vi "Test.Runner.kria.bats.parser.vi"() -> ()   [LabVIEW 2020]
uses:
  <vilib>/rvi/interface/nirviOpenFPGA/nirviOpenFPGA.xnode
  <vilib>/rvi/interface/nirviMethod/nirviMethod.xnode
  <vilib>/rvi/interface/nirviCloseFPGA/nirviCloseFPGA.xnode
  <vilib>/rvi/errors/niLvFpgaMergeErrorWithErrorCode.vi
  <vilib>/FPGAPlugInAG/Dynamic/niLvFpga_ReadFifo_Dynamic.vi
  <vilib>/rvi/interface/nirviReadWriteControl/nirviReadWriteControl.xnode
  <vilib>/rvi/interface/Simulation/niFpgaSimulationCallBeginRW.vi
  <vilib>/rvi/errors/niLvFpgaAdjustHostInterfaceError.vi
  submodules/Market.Data.Common/host/fpganow.common.host.lvlib
  NiFpgaLv.dll
  <vilib>/Utility/error.llb/Error Cluster From Error Code.vi
  <vilib>/FPGAPlugInAG/Dynamic/niLvFpga_Run_Dynamic.vi
  <vilib>/FPGAPlugInAG/Dynamic/niLvFpga_WriteFifo_Dynamic.vi
  <vilib>/FPGAPlugInAG/Dynamic/niLvFpga_Close_Dynamic.vi
  FPGA Bitfiles/market.data.poc_FPGATarget_poc.ip.kria_VbtSJiBgbQ0.lvbitx
  fpga/poc.ip.kria.vi
  <vilib>/FPGAPlugInAG/USRP-X410/niLvFpga_Open_USRP-X410.vi
  <vilib>/rvi/interface/common/dynamic/niFpgaDynamicAddResources.vi
  submodules/Market.Data.Common/fpga/orderbook.command.type.ctl
  submodules/Market.Data.Common/fpga/fpganow.common.fpga.lvlib
  submodules/Market.Data.Common/fpga/orderbook.command.ctl
panel:
  out "MDebug":u64[][](array[numeric]) format="%.0x"
  out "Ob.cmd [str]":string[](array[string])
  out "Data Sent 3":u64[][](array[numeric]) format="%016x"
  out "Debug":u64[][](array[numeric]) format="%.0x"
  out "Deserialized\nOrderBook.Commands":u64[](array[numeric]) format="%.0x"
  out "OrderBook.Command[]":T1[](array[typedef]) {"price" format="%.0x"; "symbol" format="%.0x"; "orderId" format="%.0x"; "side" format="%.0x"}
  out "error out":errorcluster
  in  "error in":errorcluster
  in  "Raw_Data File Path":path=path "C:/work/fpganow/Market.Data.PoC/cboe_pitch/generated_2025_05_02.pcap"
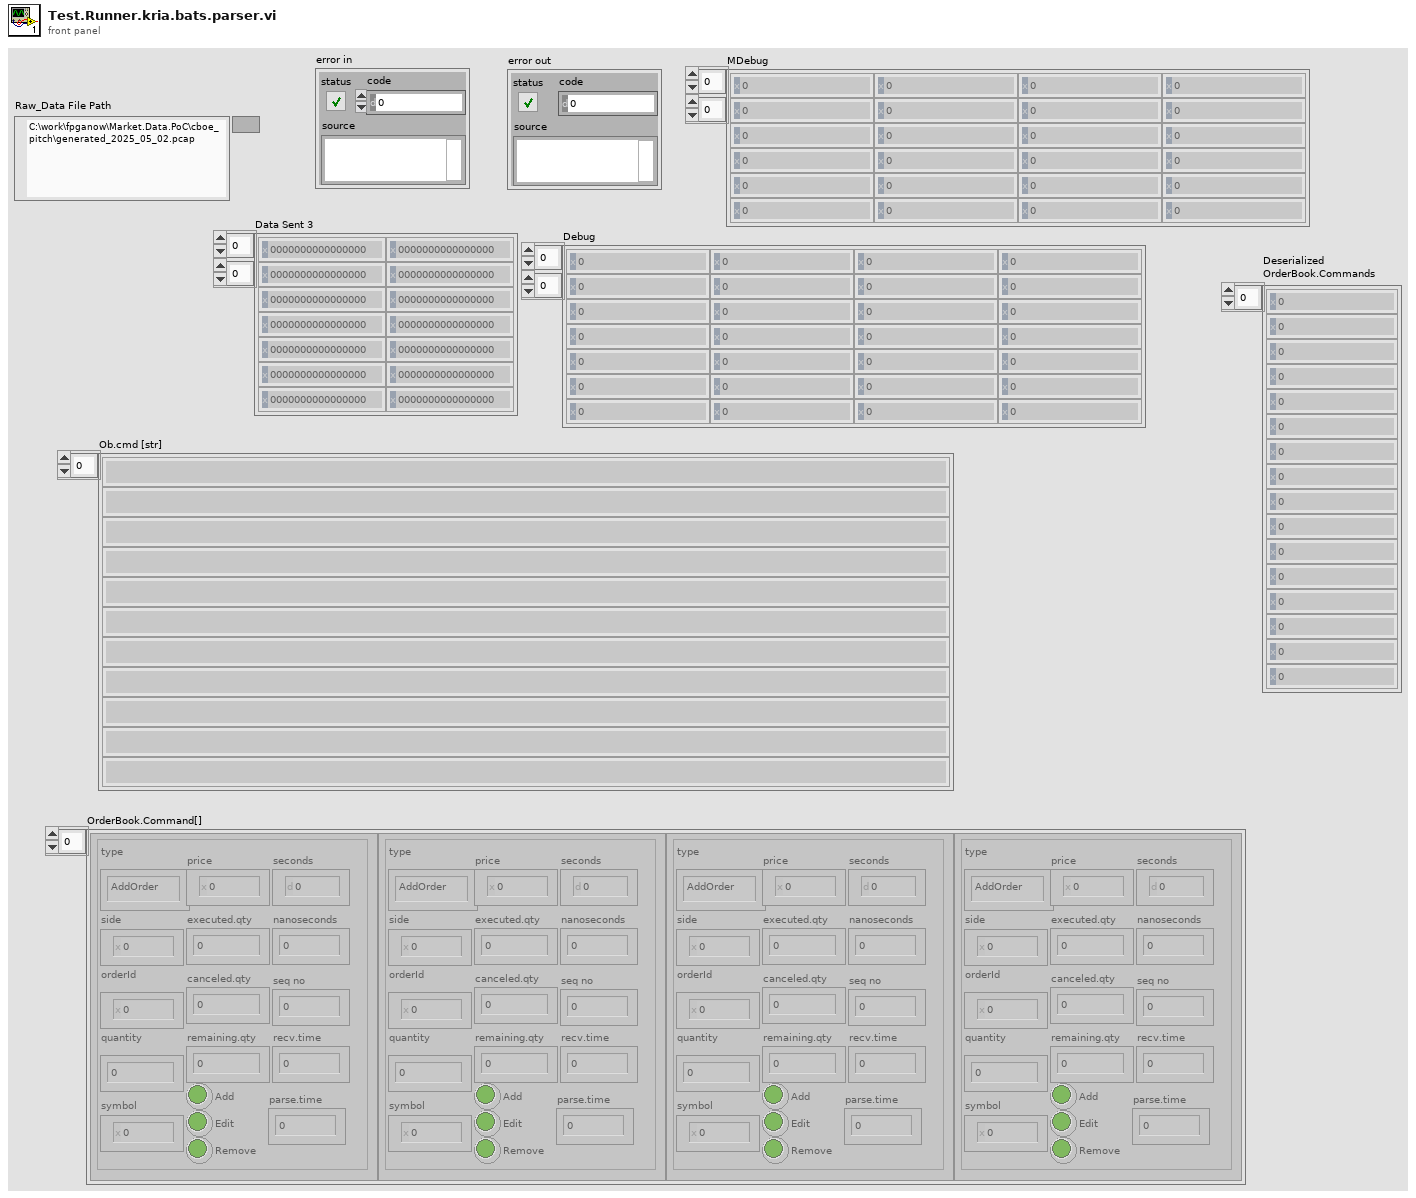
[diagram p1: front panel]
types:
  T1 = typedef "fpganow.common.fpga.lvlib/orderbook.command.ctl" = cluster{"type":T2, "side":u8, "orderId ":u64, "quantity":u32, "symbol":u64, "price":u64, "executed.qty":u32, "canceled.qty":u32, "remaining.qty":u32, "seconds":u64, "nanoseconds":u64, "Add":bool, "Edit":bool, "Remove":bool, "seq no":u32, "recv.time":u64, "parse.time":u64}
  T2 = typedef "fpganow.common.fpga.lvlib/orderbook.command.type.ctl" = enum8{"Time", "AddOrder", "OrderExecuted", "OrderExecutedAtPrice", "ReduceSize", "ModifyOrder", "DeleteOrder", "Get.Everything", "Get.All.Orders", "Get.Top"}
  T3 = typedef "record.ctl" = cluster{"ts_sec":u32, "ts_usec":u32, "incl_len":u32, "orig_len":u32, "payload":u8[]}
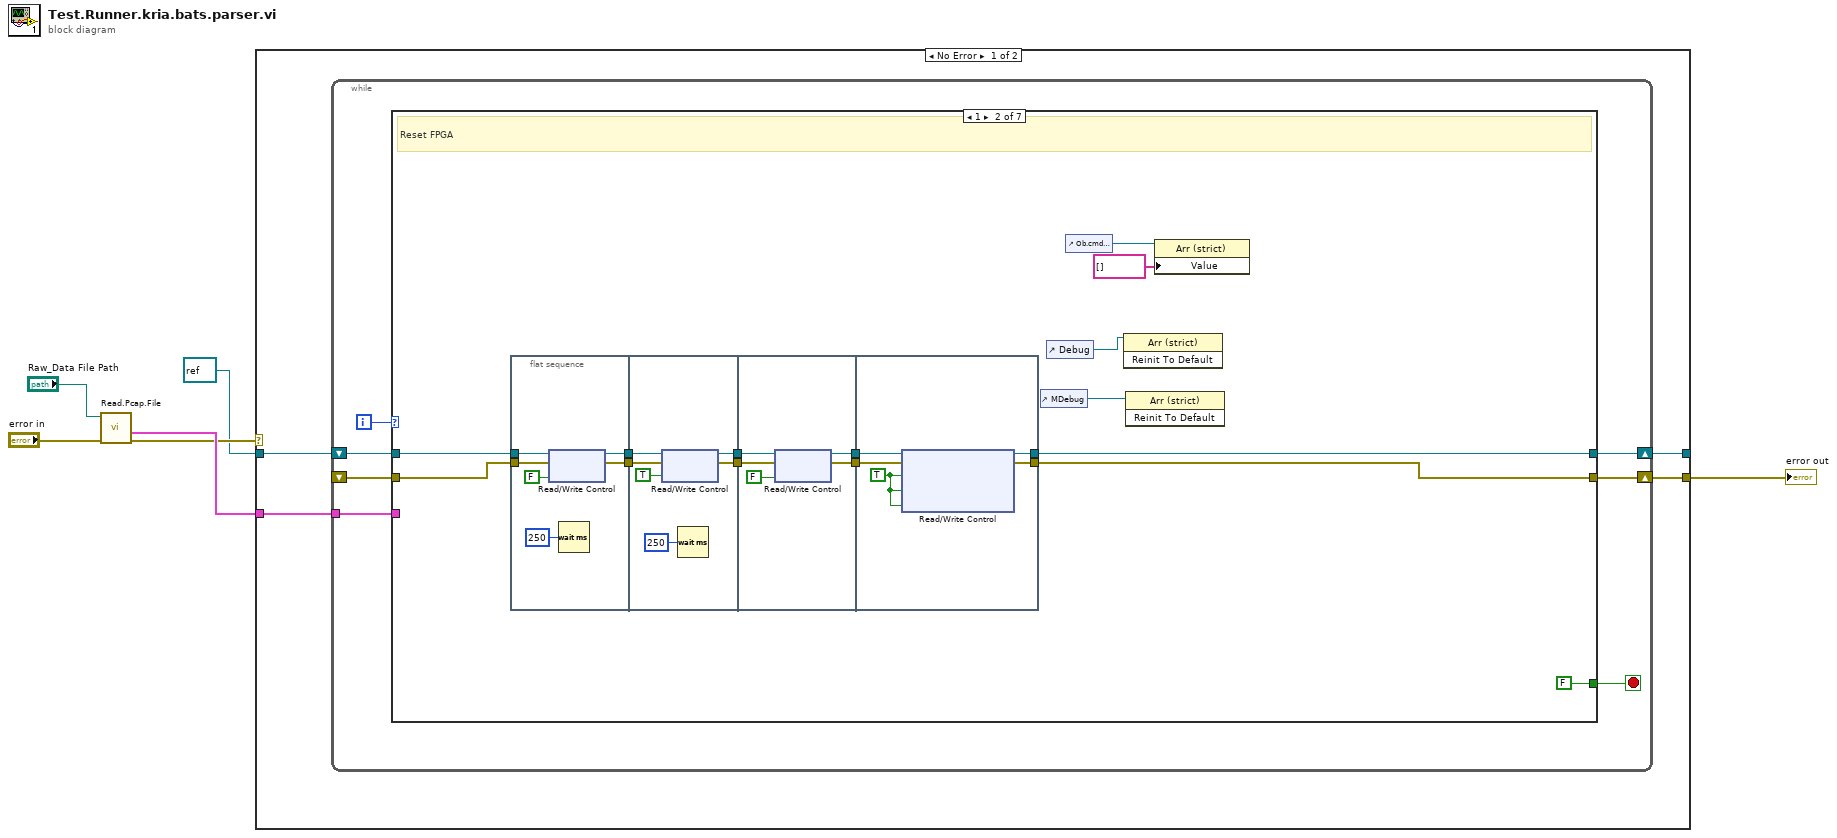
[diagram p0: block diagram]
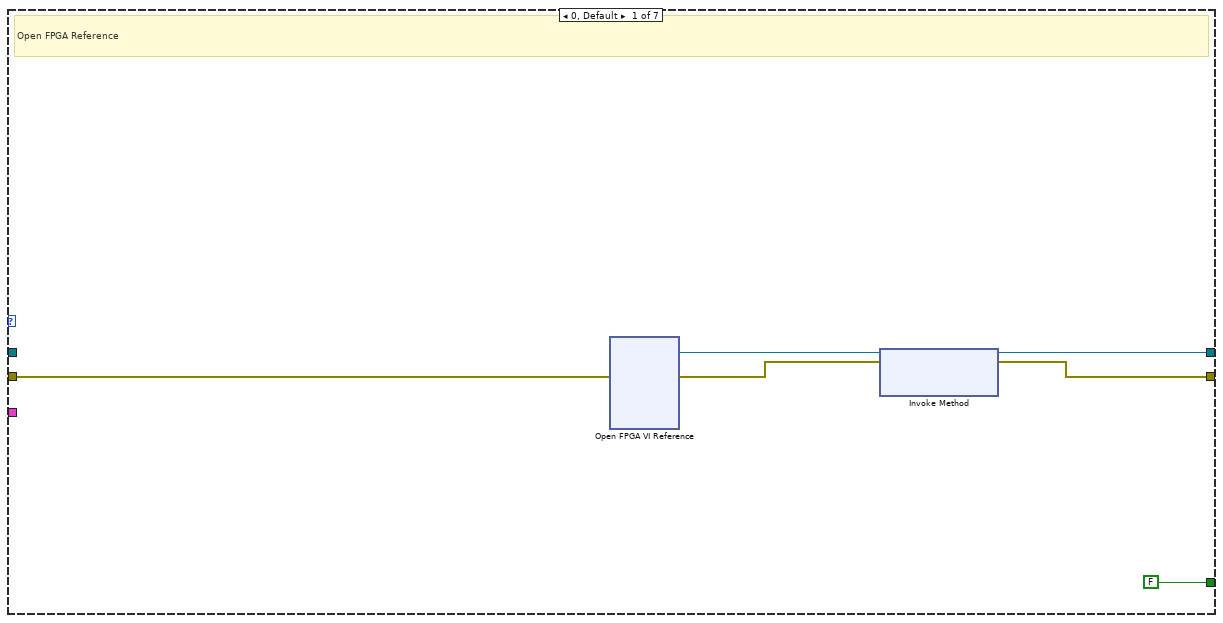
[diagram p2: hidden frame]
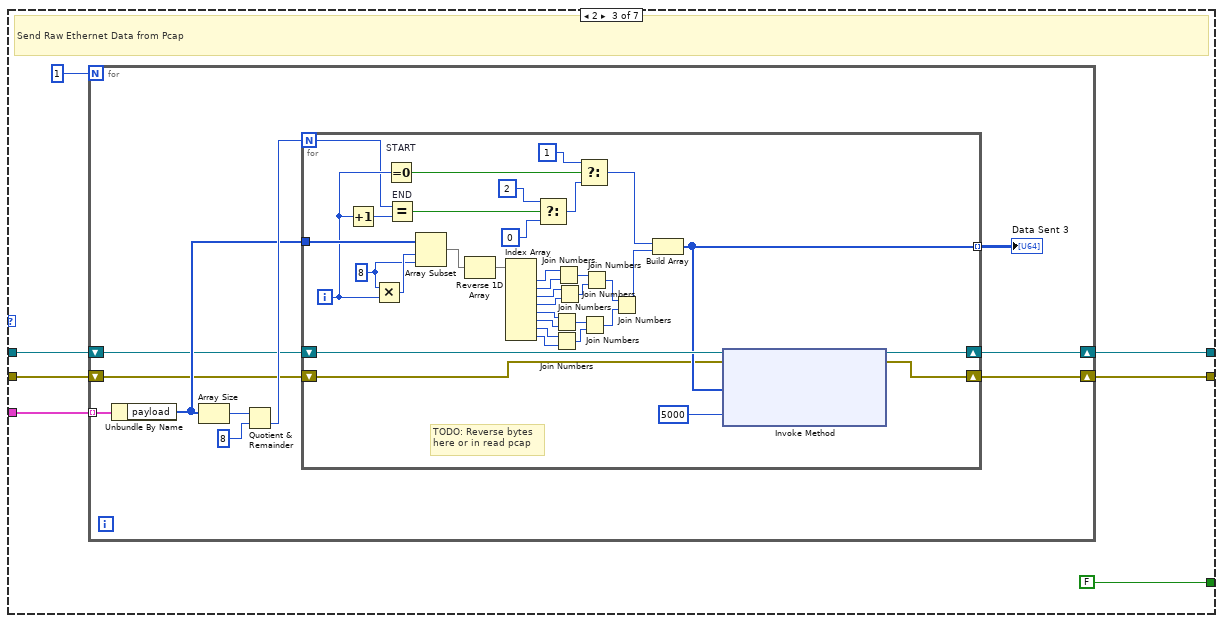
[diagram p3: hidden frame]
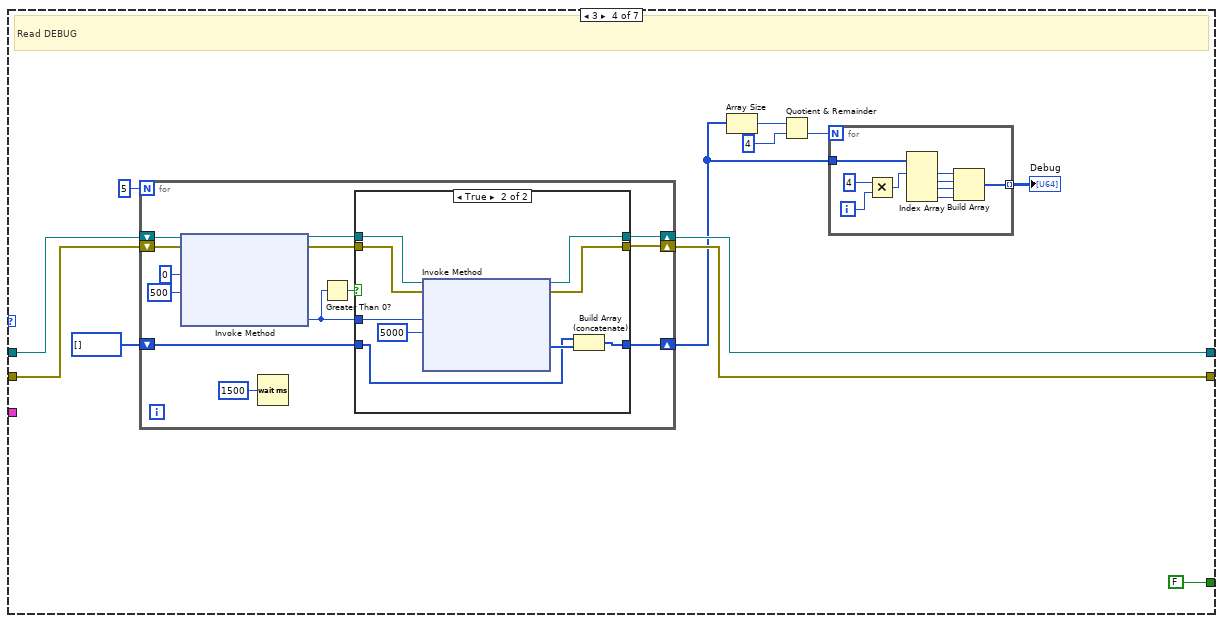
[diagram p4: hidden frame]
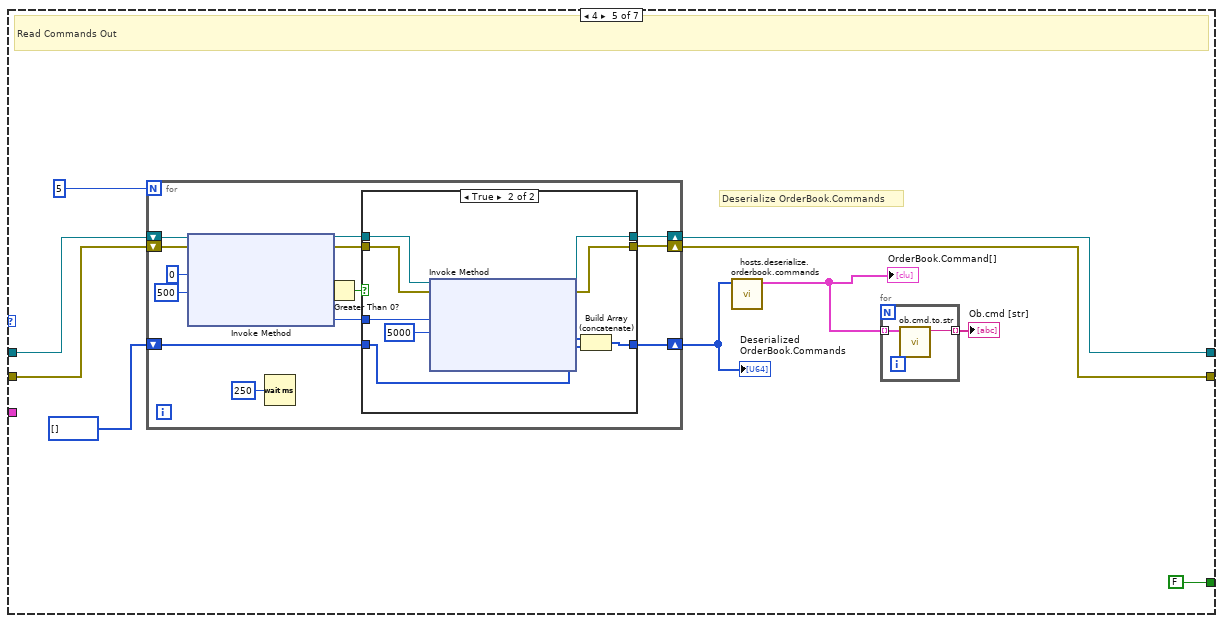
[diagram p6: hidden frame]
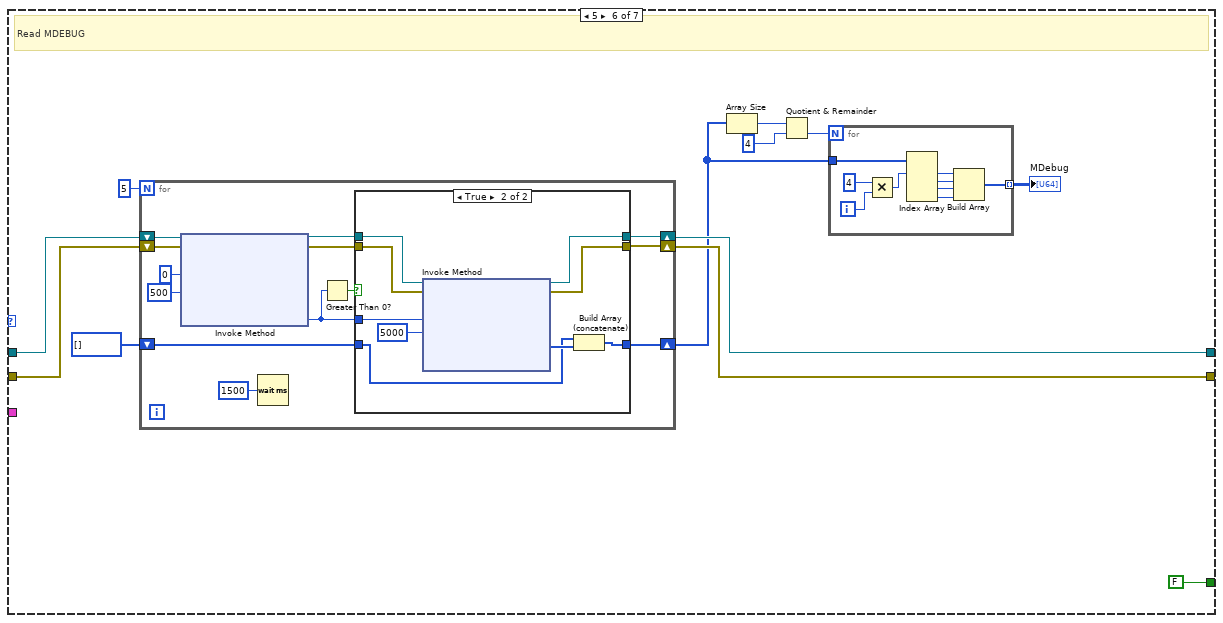
[diagram p8: hidden frame]
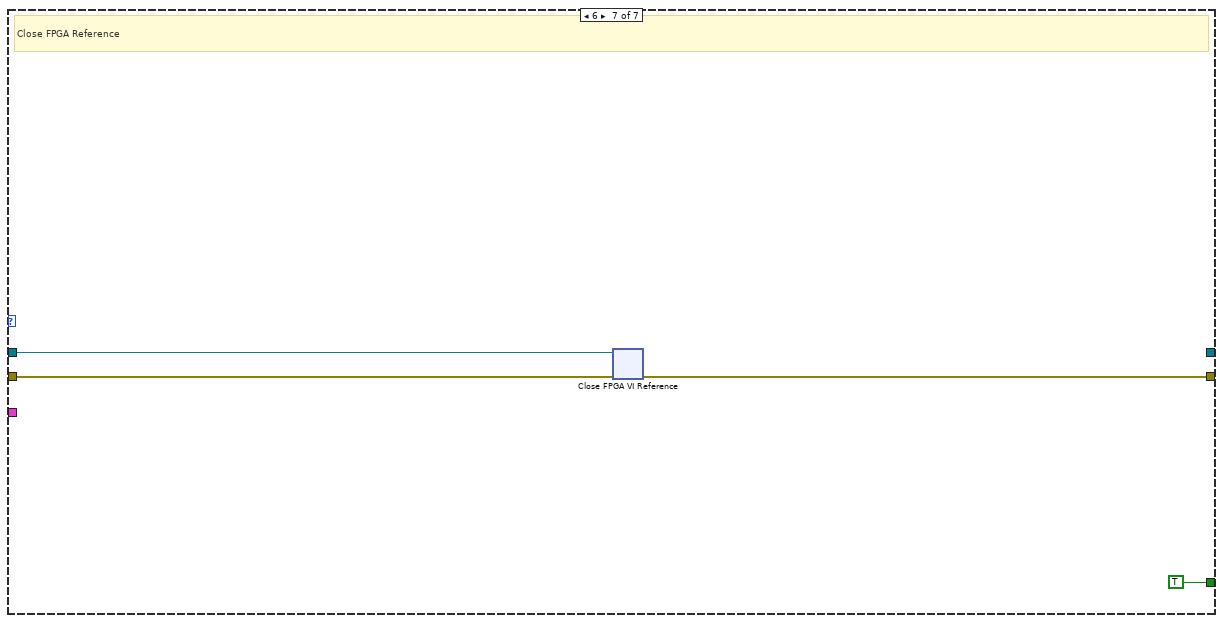
[diagram p10: hidden frame]
diagram:
  n1 = call "Read.Pcap.File.vi"("error in"="error in", "Path"="Raw_Data File Path") -> ("error out"=w4:errorcluster, "Records"=w5:T3[])  [unwired: 6 in, 2 out]
  n2 = case shown="No Error" w4 {
    selector: w4 -> [_ w247]
    tunnel: w5 -> [w10 _]
    tunnel: refnum<k20> refnum ("FPGA VI Reference Out") -> [w9 _]
    tunnel: [w8 _] -> _
    tunnel: [w7 w247] -> w3
    frame No Error {
      n3 = while {
        tunnel: w10 -> [w17]
        shift-right: [w11] -> w8
        shift-left: w9 -> [w16]
        shift-right: [w15] -> w7
        shift-left: _ -> [w14]
        i -> [w13]
        stop <- w12 stop-if-true
        n4 = case shown="1" w13 {
          tunnel: w17 -> [_ _ w62 _ _ _ _]
          tunnel: w16 -> [_ w38 w67 w125 w168 w208 w246]
          tunnel: [w19 w37 w66 w122 w165 w205 _] -> w11
          tunnel: [w18 w36 w65 w121 w164 w204 w244] -> w15
          tunnel: w14 -> [w22 w35 w64 w123 w166 w206 w245]
          tunnel: [FALSE FALSE FALSE FALSE FALSE FALSE TRUE] -> w12
          frame 0, Default {
            # "Open FPGA Reference"
            n5 = xnode "Open FPGA VI Reference"("error in"=w22) -> ("FPGA VI Reference Out"=w21:refnum<k20>, "error out"=w20:errorcluster)  [unwired: 1 in]
            n6 = xnode "Invoke Method"("FPGA VI Reference In"=w21, "error in"=w20) -> ("FPGA VI Reference Out"=w19:refnum<k20>, "error out"=w18:errorcluster)  [unwired: 1 in]
          }
          frame 1 {
            # "Reset FPGA"
            n7 = flat-sequence {
              tunnel: w38 -> [w44]
              tunnel: w35 -> [w41]
              tunnel: [w43] -> w33
              tunnel: [w42] -> w32
              tunnel: w33 -> [w49]
              tunnel: w32 -> [w50]
              tunnel: [w47] -> w31
              tunnel: [w48] -> w30
              tunnel: w31 -> [w54]
              tunnel: w30 -> [w55]
              tunnel: [w52] -> w25
              tunnel: [w53] -> w24
              tunnel: [w58] -> w36
              tunnel: [w57] -> w37
              tunnel: w25 -> [w59]
              tunnel: w24 -> [w60]
              frame #0 {
                n8 = xnode "Read/Write Control"("FPGA VI Reference In"=w44, "error in"=w41, "ip.reset"=FALSE ("Reset")) -> ("FPGA VI Reference Out"=w43:refnum<k20>, "error out"=w42:errorcluster)
                n9 = Wait (ms)(milliseconds to wait=u32 250) -> ()  [unwired: 1 out]
              }
              frame #1 {
                n10 = xnode "Read/Write Control"("FPGA VI Reference In"=w49, "error in"=w50, "ip.reset"=TRUE ("Reset")) -> ("FPGA VI Reference Out"=w47:refnum<k20>, "error out"=w48:errorcluster)
                n11 = Wait (ms)(milliseconds to wait=u32 250) -> ()  [unwired: 1 out]
              }
              frame #2 {
                n12 = xnode "Read/Write Control"("FPGA VI Reference In"=w54, "error in"=w55, "ip.reset"=FALSE ("Reset")) -> ("FPGA VI Reference Out"=w52:refnum<k20>, "error out"=w53:errorcluster)
              }
              frame #3 {
                w56 = TRUE ("MDEBUG.TREADY")
                n13 = xnode "Read/Write Control"("FPGA VI Reference In"=w59, "error in"=w60, "MDEBUG.TREADY"=w56, "CMD.TREADY"=w56, "DEBUG.TREADY"=w56) -> ("FPGA VI Reference Out"=w57:refnum<k20>, "error out"=w58:errorcluster)
              }
            }
            n14 = control-ref of="MDebug"() -> (w29:refnum<vi>)
            n15 = control-ref of="Debug"() -> (w28:refnum<vi>)
            n16 = control-ref of="Ob.cmd [str]"() -> (w27:refnum<vi>)
            n17 = invoke class="Arr (strict)" method="Reinit To Default"(reference=w28) -> ()  [unwired: 2 in, 3 out]
            n18 = invoke class="Arr (strict)" method="Reinit To Default"(reference=w29) -> ()  [unwired: 2 in, 3 out]
            n19 = property class="Arr (strict)"(reference=w27, "Value"=string[] []) -> ()  [unwired: 1 in, 2 out]
          }
          frame 2 {
            # "Send Raw Ethernet Data from Pcap"
            n20 = for {
              N: 1 -> [_]
              tunnel: w62 -> [w73] mode=indexing
              shift-right: [w71] -> w66
              shift-left: w67 -> [w70]
              shift-right: [w69] -> w65
              shift-left: w64 -> [w68]
              n21 = Unbundle By Name(w73) -> ("payload"=w74:u8[])
              n22 = Array Size(array=w74) -> (size(s)=w77:i32)
              n23 = Quotient & Remainder(x=w77, y=8) -> (floor(x/y)=w75:i32)  [unwired: 1 out]
              n24 = for {
                N: w75 -> [w109]
                tunnel: w74 -> [w111]
                tunnel: [w83] -> w72 mode=indexing
                shift-right: [w85] -> w71
                shift-left: w70 -> [w84]
                shift-right: [w81] -> w69
                shift-left: w68 -> [w80]
                i -> [w110]
                w112 = 8 ("x")
                # "TODO: Reverse bytes\nhere or in read pcap"
                n25 = Increment(x=w110) -> (x+1=w108:i32)
                n26 = Multiply(x=w112, y=w110) -> (x*y=w113:i32)
                n27 = Equal To 0? "START"(x=w110) -> (x = 0?=w107:bool)
                n28 = Equal? "END"(x=w109, y=w108) -> (x = y?=w105:bool)
                n29 = Array Subset(array=w111, index=w113, length=w112) -> (w78:u8[])
                n30 = Reverse 1D Array(array=w78) -> (reversed array=w79:u8[])
                n31 = Index Array(array=w79) -> (element #1=w100:u8, element #2=w101:u8, element #3=w99:u8, element #4=w98:u8, element #5=w96:u8, element #6=w97:u8, element #7=w95:u8, element #8=w94:u8)  [unwired: 8 in]
                n32 = Select(t=u64 2, s=w105, f=u64 0) -> (s? t:f=w102:u64)
                n33 = Join Numbers(hi=w96, lo=w97) -> ((hi.lo)=w91:u16)
                n34 = Join Numbers(hi=w95, lo=w94) -> ((hi.lo)=w90:u16)
                n35 = Join Numbers(hi=w100, lo=w101) -> ((hi.lo)=w93:u16)
                n36 = Join Numbers(hi=w99, lo=w98) -> ((hi.lo)=w92:u16)
                n37 = Select(t=u64 1, s=w107, f=w102) -> (s? t:f=w86:u64)
                n38 = Join Numbers(hi=w91, lo=w90) -> ((hi.lo)=w88:u32)
                n39 = Join Numbers(hi=w93, lo=w92) -> ((hi.lo)=w89:u32)
                n40 = Join Numbers(hi=w89, lo=w88) -> ((hi.lo)=w87:u64)
                n41 = Build Array(w86, w87) -> (w83:u64[])
                n42 = xnode "Invoke Method"("FPGA VI Reference In"=w84, "error in"=w80, "Data"=w83, "Timeout (ms)"=5000) -> ("FPGA VI Reference Out"=w85:refnum<k20>, "error out"=w81:errorcluster)  [unwired: 1 out]
              }
              "Data Sent 3" <- w72
            }
          }
          frame 3 {
            # "Read DEBUG"
            n43 = for {
              N: 5 -> [_]
              shift-right: [w141] -> w122
              shift-left: w125 -> [w147]
              shift-right: [w140] -> w121
              shift-left: w123 -> [w146]
              shift-right: [w142] -> w117
              shift-left: u64[] [] -> [w136]
              n44 = xnode "Invoke Method"("FPGA VI Reference In"=w147, "error in"=w146, "Number of Elements"=u32 0, "Timeout (ms)"=500) -> ("FPGA VI Reference Out"=w139:refnum<k20>, "error out"=w138:errorcluster, "Elements Remaining"=w137:u32)  [unwired: 1 out]
              n45 = Wait (ms)(milliseconds to wait=u32 1500) -> ()  [unwired: 1 out]
              n46 = Greater Than 0?(x=w137) -> (x > 0?=w143:bool)
              n47 = case shown="True" w143 {
                tunnel: [w148 w158] -> w142
                tunnel: [w150 w157] -> w141
                tunnel: [w149 w156] -> w140
                tunnel: w139 -> [w150 w155]
                tunnel: w138 -> [w149 w154]
                tunnel: w137 -> [_ w153]
                tunnel: w136 -> [w148 w151]
                frame False {
                }
                frame True {
                  n48 = xnode "Invoke Method"("FPGA VI Reference In"=w155, "error in"=w154, "Number of Elements"=w153, "Timeout (ms)"=5000) -> ("FPGA VI Reference Out"=w157:refnum<k20>, "error out"=w156:errorcluster, "Data"=w159:u64[])  [unwired: 1 out]
                  n49 = Build Array (concatenate)(w151, w159) -> (w158:u64[])
                }
              }
            }
            n50 = Array Size(array=w117) -> (size(s)=w119:i32)
            n51 = Quotient & Remainder(x=w119, y=4) -> (floor(x/y)=w115:i32)  [unwired: 1 out]
            n52 = for {
              N: w115 -> [_]
              tunnel: w117 -> [w134]
              tunnel: [w126] -> w116 mode=indexing
              i -> [w133]
              n53 = Multiply(x=4, y=w133) -> (x*y=w132:i32)
              n54 = Index Array(array=w134, index #1=w132) -> (element #1=w130:u64, element #2=w127:u64, element #3=w128:u64, element #4=w129:u64)  [unwired: 3 in]
              n55 = Build Array(w130, w127, w128, w129) -> (w126:u64[])
            }
            "Debug" <- w116
          }
          frame 4 {
            # "Deserialize OrderBook.Commands"
            # "Read Commands Out"
            n56 = for {
              N: 5 -> [_]
              shift-right: [w178] -> w165
              shift-left: w168 -> [w184]
              shift-right: [w177] -> w164
              shift-left: w166 -> [w183]
              shift-right: [w179] -> w162
              shift-left: u64[] [] -> [w173]
              n57 = xnode "Invoke Method"("FPGA VI Reference In"=w184, "error in"=w183, "Number of Elements"=u32 0, "Timeout (ms)"=500) -> ("FPGA VI Reference Out"=w176:refnum<k20>, "error out"=w175:errorcluster, "Elements Remaining"=w174:u32)  [unwired: 1 out]
              n58 = Wait (ms)(milliseconds to wait=u32 250) -> ()  [unwired: 1 out]
              n59 = Greater Than 0?(x=w174) -> (x > 0?=w180:bool)
              n60 = case shown="True" w180 {
                tunnel: [w185 w195] -> w179
                tunnel: [w187 w194] -> w178
                tunnel: [w186 w193] -> w177
                tunnel: w176 -> [w187 w192]
                tunnel: w175 -> [w186 w191]
                tunnel: w174 -> [_ w190]
                tunnel: w173 -> [w185 w188]
                frame False {
                }
                frame True {
                  n61 = xnode "Invoke Method"("FPGA VI Reference In"=w192, "error in"=w191, "Number of Elements"=w190, "Timeout (ms)"=5000) -> ("FPGA VI Reference Out"=w194:refnum<k20>, "error out"=w193:errorcluster, "Data"=w196:u64[])  [unwired: 1 out]
                  n62 = Build Array (concatenate)(w188, w196) -> (w195:u64[])
                }
              }
            }
            "Deserialized\nOrderBook.Commands" <- w162
            n63 = call "hosts.deserialize.orderbook.commands.vi"("DataIn"=w162) -> ("OrderBook.Command[]"=w160:T1[])  [unwired: 10 in]
            "OrderBook.Command[]" <- w160
            n64 = for {
              tunnel: w160 -> [w171] mode=indexing
              tunnel: [w170] -> w161 mode=indexing
              n65 = call "ob.cmd.to.str.vi"("orderbook.command"=w171) -> ("string"=w170:string)  [unwired: 10 in]
            }
            "Ob.cmd [str]" <- w161
          }
          frame 5 {
            # "Read MDEBUG"
            n66 = for {
              N: 5 -> [_]
              shift-right: [w224] -> w205
              shift-left: w208 -> [w230]
              shift-right: [w223] -> w204
              shift-left: w206 -> [w229]
              shift-right: [w225] -> w200
              shift-left: u64[] [] -> [w219]
              n67 = xnode "Invoke Method"("FPGA VI Reference In"=w230, "error in"=w229, "Number of Elements"=u32 0, "Timeout (ms)"=500) -> ("FPGA VI Reference Out"=w222:refnum<k20>, "error out"=w221:errorcluster, "Elements Remaining"=w220:u32)  [unwired: 1 out]
              n68 = Wait (ms)(milliseconds to wait=u32 1500) -> ()  [unwired: 1 out]
              n69 = Greater Than 0?(x=w220) -> (x > 0?=w226:bool)
              n70 = case shown="True" w226 {
                tunnel: [w231 w241] -> w225
                tunnel: [w233 w240] -> w224
                tunnel: [w232 w239] -> w223
                tunnel: w222 -> [w233 w238]
                tunnel: w221 -> [w232 w237]
                tunnel: w220 -> [_ w236]
                tunnel: w219 -> [w231 w234]
                frame False {
                }
                frame True {
                  n71 = xnode "Invoke Method"("FPGA VI Reference In"=w238, "error in"=w237, "Number of Elements"=w236, "Timeout (ms)"=5000) -> ("FPGA VI Reference Out"=w240:refnum<k20>, "error out"=w239:errorcluster, "Data"=w242:u64[])  [unwired: 1 out]
                  n72 = Build Array (concatenate)(w234, w242) -> (w241:u64[])
                }
              }
            }
            n73 = Array Size(array=w200) -> (size(s)=w202:i32)
            n74 = Quotient & Remainder(x=w202, y=4) -> (floor(x/y)=w198:i32)  [unwired: 1 out]
            n75 = for {
              N: w198 -> [_]
              tunnel: w200 -> [w217]
              tunnel: [w209] -> w199 mode=indexing
              i -> [w216]
              n76 = Multiply(x=4, y=w216) -> (x*y=w215:i32)
              n77 = Index Array(array=w217, index #1=w215) -> (element #1=w213:u64, element #2=w210:u64, element #3=w211:u64, element #4=w212:u64)  [unwired: 3 in]
              n78 = Build Array(w213, w210, w211, w212) -> (w209:u64[])
            }
            "MDebug" <- w199
          }
          frame 6 {
            # "Close FPGA Reference"
            n79 = xnode "Close FPGA VI Reference"("FPGA VI Reference In"=w246, "error in"=w245) -> ("error out"=w244:errorcluster)
          }
        }
      }
    }
    frame Error {
    }
  }
  "error out" <- w3
